vi "flatten PID.vi"(11 "PID Loop":T1={"ID"="", "Setpoint"=refnum, "Process Variable"=refnum, "Output"=refnum, "PID gains"={"proportional gain (Kc)"=1.0, "integral time (Ti, min)"=0.01, "derivative time (Td, min)"=0.0}, "output range"={"output high"=100.0, "output low"=-100.0}} {"output range"."output low" format="%.2f"; "output range"."output high" format="%.2f"}) -> (3 "String":string)   [LabVIEW 2014, in "Tagbus PID Module configuration.lvclass"]
doc: "This VI flattens a PID Loop to a string so that the object can be saved to a file."
uses:
  Tagbus PID Module configuration.lvclass
  <vilib>/NI/Tag Bus Module Framework/channel/TBM channel.lvclass
  <vilib>/NI/Configuration Framework/serializable configuration/NISE_CEF_serializable configuration.lvclass
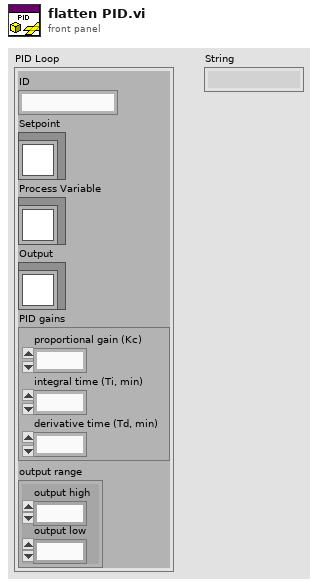
[diagram p1: front panel]
types:
  T1 = cluster{"ID":string, "Setpoint":refnum<class "TBM channel.lvclass">, "Process Variable":refnum<class "TBM channel.lvclass">, "Output":refnum<class "TBM channel.lvclass">, "PID gains":cluster{"proportional gain (Kc)":dbl, "integral time (Ti, min)":dbl, "derivative time (Td, min)":dbl}, "output range":cluster{"output high":dbl, "output low":dbl}}
  T2 = cluster{"proportional gain (Kc)":dbl, "integral time (Ti, min)":dbl, "derivative time (Td, min)":dbl}
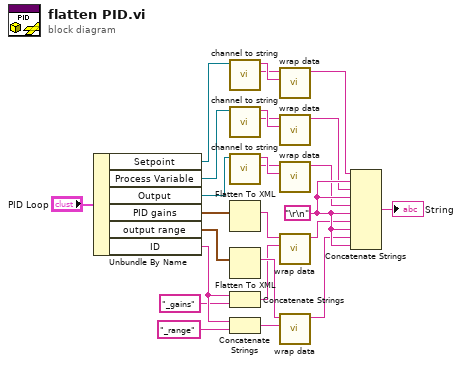
[diagram p0: block diagram]
diagram:
  w26 = "\r\n"
  n1 = Unbundle By Name("PID Loop") -> ("Setpoint"=w4:refnum<class "TBM channel.lvclass">, "Process Variable"=w5:refnum<class "TBM channel.lvclass">, "Output"=w6:refnum<class "TBM channel.lvclass">, "PID gains"=w11:T2, "output range"=w12:cluster{"output high":dbl, "output low":dbl}, "ID"=w19:string)
  n2 = call <vilib>:"channel to string.vi"("channel in"=w4) -> ("channel data"=w1:string, "identifier"=w2:string)  [unwired: 9 in]
  n3 = call <vilib>:"channel to string.vi"("channel in"=w5) -> ("channel data"=w7:string, "identifier"=w8:string)  [unwired: 9 in]
  n4 = call <vilib>:"channel to string.vi"("channel in"=w6) -> ("channel data"=w9:string, "identifier"=w10:string)  [unwired: 9 in]
  n5 = Flatten To XML(anything=w11) -> (xml string=w13:string)
  n6 = Flatten To XML(anything=w12) -> (xml string=w18:string)
  n7 = Concatenate Strings(w19, "_gains" ("string")) -> (w14:string)
  n8 = Concatenate Strings(w19, "_range" ("string")) -> (w17:string)
  n9 = call <vilib>:"wrap data.vi"("identifier"=w2, "data to wrap"=w1) -> ("wrapped data"=w21:string)  [unwired: 9 in]
  n10 = call <vilib>:"wrap data.vi"("identifier"=w8, "data to wrap"=w7) -> ("wrapped data"=w22:string)  [unwired: 9 in]
  n11 = call <vilib>:"wrap data.vi"("identifier"=w10, "data to wrap"=w9) -> ("wrapped data"=w23:string)  [unwired: 9 in]
  n12 = call <vilib>:"wrap data.vi"("identifier"=w14, "data to wrap"=w13) -> ("wrapped data"=w24:string)  [unwired: 9 in]
  n13 = call <vilib>:"wrap data.vi"("identifier"=w17, "data to wrap"=w18) -> ("wrapped data"=w25:string)  [unwired: 9 in]
  n14 = Concatenate Strings(w21, w26, w22, w26, w23, w26, w24, w26, w25, w26) -> (→"String":string)
